vi "ExperimentNameCreator.vi"(11 "Experiment ID":string) -> (3 "Experiment Name":string)   [LabVIEW 2013]
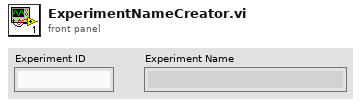
[diagram p1: front panel]
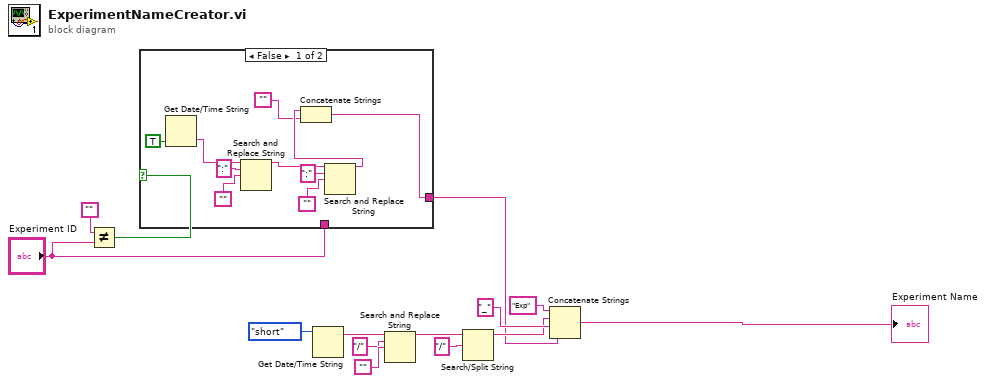
[diagram p0: block diagram]
diagram:
  n1 = Not Equal?(x="", y="Experiment ID") -> (x != y?=w3:bool)
  n2 = case shown="False" w3 {
    tunnel: "Experiment ID" -> [_ w25]
    tunnel: [w21 w25] -> w1
    frame False {
      n3 = Get Date/Time String(want seconds? (F)=TRUE) -> (time string=w24:string)  [unwired: 2 in, 1 out]
      n4 = Search and Replace String(input string=w24, search string=":", replace string="") -> (result string=w20:string)  [unwired: 5 in, 3 out]
      n5 = Search and Replace String(input string=w20, search string=":", replace string="") -> (result string=w18:string)  [unwired: 5 in, 3 out]
      n6 = Concatenate Strings(w18, "") -> (w21:string)
    }
    frame True {
    }
  }
  n7 = Get Date/Time String(date format (0)=enum16{"short", "long", "abbreviated"}."short") -> (date string=w7:string)  [unwired: 2 in, 1 out]
  n8 = Search and Replace String(input string=w7, search string="/", replace string="") -> (result string=w11:string)  [unwired: 5 in, 3 out]
  n9 = Search/Split String(string=w11, search string/char (-)="/" ("search string")) -> (substring before match=w2:string)  [unwired: 1 in, 2 out]
  n10 = Concatenate Strings("Exp" ("string"), w2, "_" ("string"), w1) -> (→"Experiment Name":string)
